vi "set_thermocouple_calibration_type.vi"(8 "error in (no error)":errorcluster, 10 "Thermocouple calibration type":T1="0", 11 "connection ID":refnum<k5>) -> (0 "error out":errorcluster, 3 "connection ID out":refnum<k5>)   [LabVIEW 2018]
uses:
  typedefs/thermocouple_calibration_types.ctl
panel:
  out "bytes written":i32
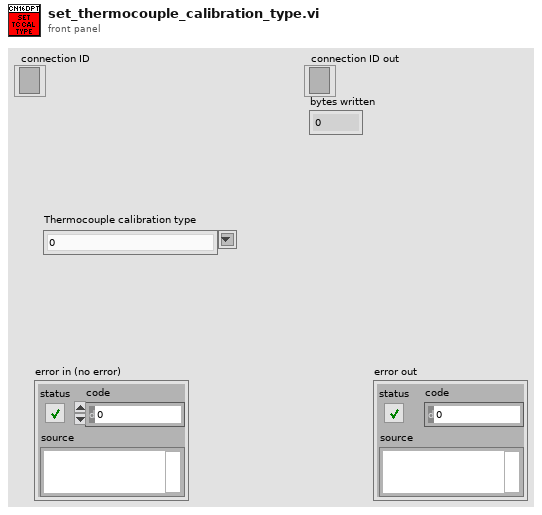
[diagram p1: front panel]
types:
  T1 = typedef "thermocouple_calibration_types.ctl" = string
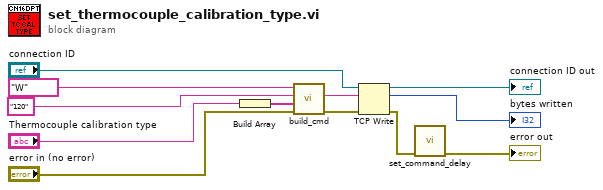
[diagram p0: block diagram]
diagram:
  n1 = Build Array("Thermocouple calibration type") -> (w6:T1[])
  n2 = call "build_cmd.vi"("error in (no error)"="error in (no error)", "Parameter list"=w6, "Command ID"="120", "Command class"="W") -> ("error out"=w9:errorcluster, "Command"=w8:string)  [unwired: 6 in]
  n3 = TCP Write(connection ID="connection ID", data in=w8, error in (no error)=w9) -> (connection ID out=→"connection ID out":refnum<k5>, bytes written=→"bytes written":i32, error out=w2:errorcluster)  [unwired: 1 in]
  n4 = call "set_command_delay.vi"("error in (no error)"=w2) -> ("error out"=→"error out":errorcluster)  [unwired: 10 in]
